vi "FSK_Pluse.vi"(8 "error in (no error)":errorcluster caption="错误输入（无错误）", 9 "pos":i32=7, 10 "RecvSig":dbl[](array[numeric]), 11 "PathIn":path) -> (0 "error out":errorcluster caption="错误输出", 2 "samplePulse":dbl[](array[numeric]) format="%#_13g", 3 "PathOut":path)   [LabVIEW 2015]
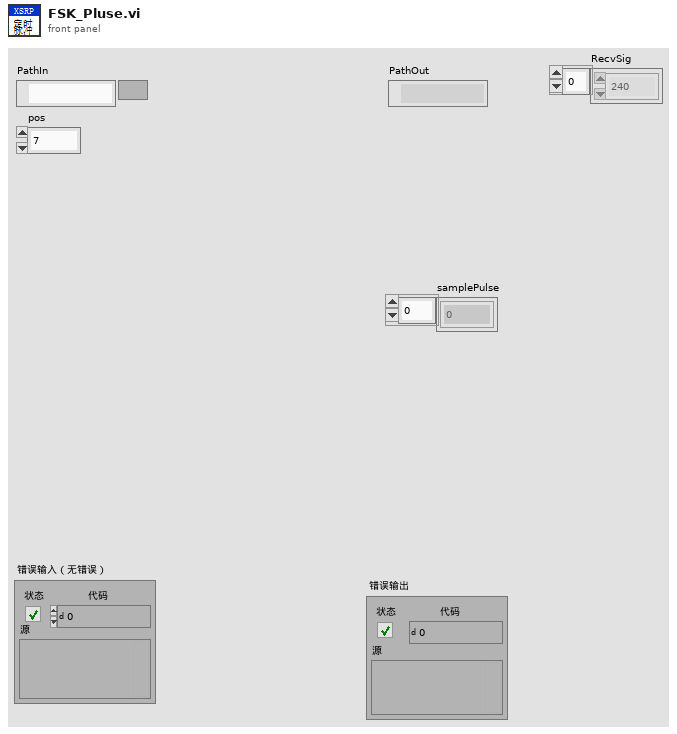
[diagram p1: front panel]
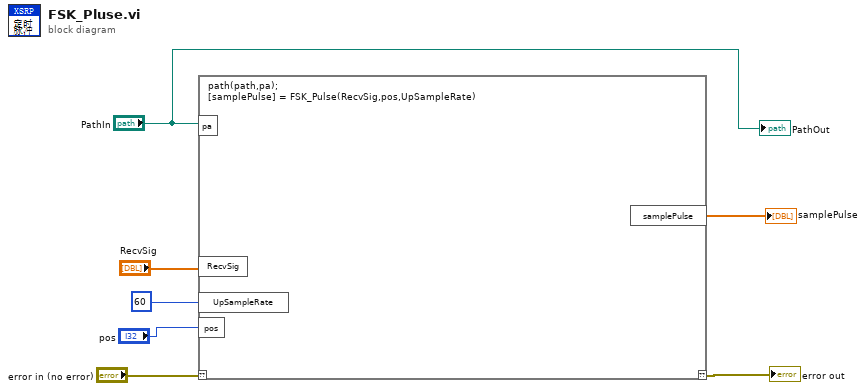
[diagram p0: block diagram]
diagram:
  n1 = script code="path(path,pa);\n[samplePulse] = FSK_Pulse(RecvSig,pos,UpSampleRate)"("??"="error in (no error)", "pa"="PathIn", "RecvSig"="RecvSig", "UpSampleRate"=60, "pos"="pos") -> ("??"=→"error out":errorcluster, "samplePulse"=→"samplePulse":dbl[])
  "PathOut" <- "PathIn"
